vi "Read Spectral Waveform.vi"(8 "error in (no error)":errorcluster, 11 "VISA resource name":refnum<visa-resource-name>) -> (0 "error out":errorcluster, 2 "Spectral Waveform":cluster{dbl[], dbl[]}(graph), 3 "VISA resource name out":refnum<visa-resource-name>)   [LabVIEW 2018, in "Ocean Optics 2000 4000.lvlib"]
doc: "Displays the spectrum vs wavelength in a waveform graph.\n\n<b>Note:</b> Do not put this VI in a loop if performance is a concern. Please see the <b>Ocean Optics 2000 4000 Acquire Continuous Waveform</b> example for an example of how to do continuous acquisition."
uses:
  Ocean Optics 2000 4000.lvlib
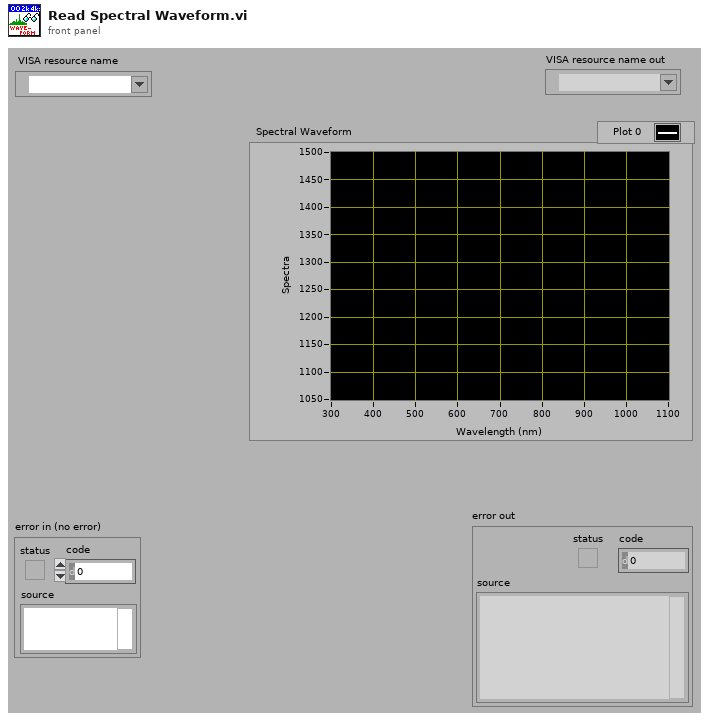
[diagram p1: front panel]
types:
  T1 = cluster{"Wavelength (nm)":dbl[], "Spectrum by Pixel Number":dbl[]}
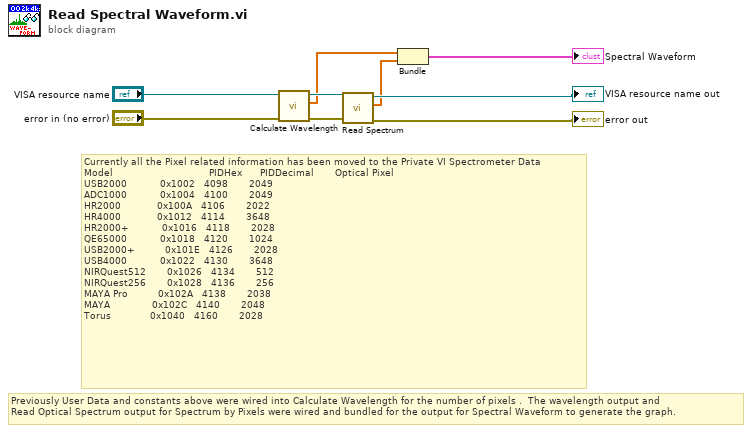
[diagram p0: block diagram]
diagram:
  # "Currently all the Pixel related information has been moved to the Private VI Spectrometer Data\nModel\t                               PIDHex     \tPIDDecimal      \tOptical Pixel\nUSB2000\t          0x1002\t  4098\t      2049\t\nADC1000\t          0x1004\t  4100\t      2049 \nHR2000\t           0x100A\t  4106\t      2022\t\nHR4000\t           0x1012\t  4114\t      3648\t\nHR2000+\t          0x1016\t  4118\t      2028\t\nQE65000\t          0x1018\t  4120\t      1024\t\nUSB2000+\t         0x101E\t  4126\t      2028\t\nUSB4000\t          0x1022\t  4130\t      3648\t\nNIRQuest512\t      0x1026\t  4134\t      512\t \nNIRQuest256 \t     0x1028\t  4136\t      256\t \nMAYA Pro\t         0x102A\t  4138\t      2038\t\nMAYA\t             0x102C\t  4140\t      2048\t\nTorus\t            0x1040\t  4160\t      2028"
  # "Previously User Data and constants above were wired into Calculate Wavelength for the number of pixels .  The wavelength output and  \nRead Optical Spectrum output for Spectrum by Pixels were wired and bundled for the output for Spectral Waveform to generate the graph."
  n1 = call "Calculate Wavelength.vi"("error in (no error)"="error in (no error)", "VISA resource name"="VISA resource name") -> ("error out"=w6:errorcluster, "Wavelength (nm)"=w2:dbl[], "VISA resource name out"=w5:refnum<visa-resource-name>)  [unwired: 7 in]
  n2 = call "Read Spectrum.vi"("error in (no error)"=w6, "VISA resource name"=w5) -> ("error out"=→"error out":errorcluster, "Spectrum by Pixel Number"=w1:dbl[], "VISA resource name out"=→"VISA resource name out":refnum<visa-resource-name>)  [unwired: 7 out]
  n3 = Bundle("Wavelength (nm)"=w2, "Spectrum by Pixel Number"=w1) -> (→"Spectral Waveform":T1)  [unwired: 1 in]
